vi "ReadI32.vi"(11 "Address":u32) -> (3 "Data":i32)   [LabVIEW 2016]
uses:
  <vilib>/rvi/Memory/Memory_Emulation/nirvimemoryFastEmulation.vi
  <vilib>/rvi/Memory/Memory_Emulation/nirvimemoryEmulation.vi
  <vilib>/rvi/Emulation/niFpgaEmulationIsFPGAContextNoSignature.vi
  <vilib>/rvi/DataTransferAndStorage/Container/Common/niFpgaContainerGetUniqueNameForEmu.vi
  <vilib>/rvi/Emulation/niFpgaProcessEmulError.vi
  <vilib>/rvi/Emulation/niFpgaSctlEmulationGetInTimedLoop.vi
  <vilib>/rvi/errors/nirviReportUnexpectedCaseInternalError (U32).vi
  <vilib>/rvi/DataTransferAndStorage/Container/Common/niFpgaContainerExecOnDevCompGetState.vi
  <vilib>/rvi/Memory/Memory_Emulation/niFpgaMemoryEmulationCacheClearOnFirstRun.vi
  <vilib>/rvi/Memory/Memory_Emulation/nirvimemoryEmulationManagerCache_MakeExclusive.vi
  <vilib>/rvi/Memory/Memory_Emulation/niFpgaMemoryEmulationValidateCache.vi
  <vilib>/rvi/Memory/Memory_Emulation/nirvimemoryEmulationManagerCache_InsertValue.vi
  <vilib>/Utility/error.llb/Clear Errors.vi
  <vilib>/rvi/Memory/Memory_Emulation/nirvimemoryEmulationManagerCache_ReleaseExclusive.vi
  <vilib>/rvi/Memory/Memory_Emulation/nirvimemoryEmulationManagerCache_GetValue.vi
  <vilib>/rvi/Memory/Memory_Emulation/nirvimemoryEmulationManagerCache_SetValue.vi
  <vilib>/rvi/Emulation/niFpgaSctlEmulationResourceMgr.vi
  <vilib>/rvi/DataTransferAndStorage/Container/XNode/niFpgaContainer.xnode
  <vilib>/rvi/Memory/Memory_Emulation/niFpgaMemoryEmulationRefIn.vi
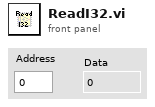
[diagram p1: front panel]
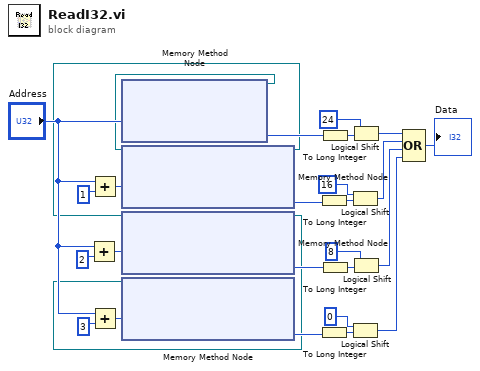
[diagram p0: block diagram]
diagram:
  n1 = Add(x="Address", y=u32 2) -> (x+y=w8:u32)
  n2 = Add(x="Address", y=u32 1) -> (x+y=w18:u32)
  n3 = Add(x="Address", y=u32 3) -> (x+y=w17:u32)
  n4 = xnode ("Memory Method Node")("Address"="Address") -> ("Data"=w27:u8, "Memory Out"=w3:refnum<k21>)  [unwired: 1 in]
  n5 = xnode ("Memory Method Node")("Address"=w18, "Memory In"=w3) -> ("Data"=w23:u8, "Memory Out"=w2:refnum<k21>)
  n6 = xnode ("Memory Method Node")("Address"=w8, "Memory In"=w2) -> ("Data"=w10:u8, "Memory Out"=w1:refnum<k21>)
  n7 = xnode ("Memory Method Node")("Address"=w17, "Memory In"=w1) -> ("Data"=w14:u8)  [unwired: 1 out]
  n8 = To Long Integer(number=w23) -> (32bit integer=w24:i32)
  n9 = To Long Integer(number=w14) -> (32bit integer=w13:i32)
  n10 = To Long Integer(number=w27) -> (32bit integer=w26:i32)
  n11 = To Long Integer(number=w10) -> (32bit integer=w11:i32)
  n12 = Logical Shift(y=i16 16, x=w24) -> (x << y=w21:i32)
  n13 = Logical Shift(y=i16 0, x=w13) -> (x << y=w5:i32)
  n14 = Logical Shift(y=i16 24, x=w26) -> (x << y=w4:i32)
  n15 = Logical Shift(y=i16 8, x=w11) -> (x << y=w6:i32)
  n16 = Compound Arithmetic op=OR(w4, w21, w6, w5) -> (→"Data":i32)
